vi "Withdrawal.vi"(8 "error in (no error)":errorcluster, 11 "ATM Controller in":refnum<class "ATM Controller.lvclass">) -> (0 "error out":errorcluster, 3 "ATM Controller out":refnum<class "ATM Controller.lvclass">)   [LabVIEW 2019, in "ATM Controller.lvlib" / "ATM Controller.lvclass"]
uses:
  ATM Controller.lvclass
  C:/Program Files (x86)/National Instruments/LabVIEW 2019/vi.lib/ActorFramework/Actor/Actor.lvclass
  <vilib>/ActorFramework/Actor/Actor.lvclass/Actor.ctl
  <vilib>/ActorFramework/Message Enqueuer/Message Enqueuer.lvclass/Message Enqueuer.ctl
  ATM Controller.lvclass/ATM Controller.ctl
  Message Name.ctl
  Simulated Configuration Database Actor/Configuration Database Actor Messages/Write Record Msg/Write Record Msg.lvclass/Write Record Msg.ctl
  ATM Controller Messages/Set ATM Message Msg/Set ATM Message Msg.lvclass/Set ATM Message Msg.ctl
  <vilib>/ActorFramework/Message Enqueuer/Init from Existing Queue.vi
  <vilib>/ActorFramework/Message Enqueuer/Enqueue.vi
  Simulated Configuration Database Actor/Configuration Database Actor Messages/Write Record Msg/Write Record Msg.lvclass
  C:/Program Files (x86)/National Instruments/LabVIEW 2019/vi.lib/ActorFramework/Message/Message.lvclass
  ATM Controller Messages/Set ATM Message Msg/Set ATM Message Msg.lvclass
  <vilib>/ActorFramework/Message Priority Queue/Priority Enqueue.vi
  <vilib>/ActorFramework/Message Enqueuer/Message Enqueuer.lvclass
  <vilib>/ActorFramework/Actor/Actor.lvclass
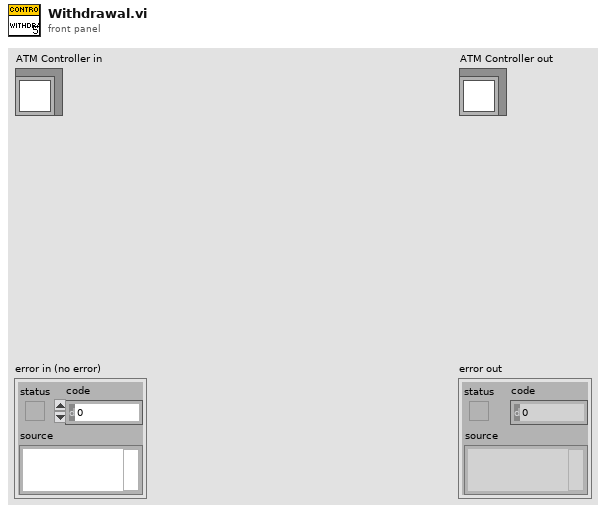
[diagram p1: front panel]
types:
  T1 = typedef "ATM Controller.lvlib/ATM Controller.lvclass/Message Name.ctl" = enum16{"Welcome", "Login", "Idle", "Invalid Login", "Terminate Session", "Deposit", "Withdrawal", "Fast Cash $50", "Withdrawal Failed", "Balance Inquiry"}
  T2 = typedef "Configuration Database Actor.lvlib/Configuration Database Actor.lvclass/Records -cluster.ctl" = cluster{"Account Number":i32, "First Name":string, "Last Name":string, "Balance":i32}
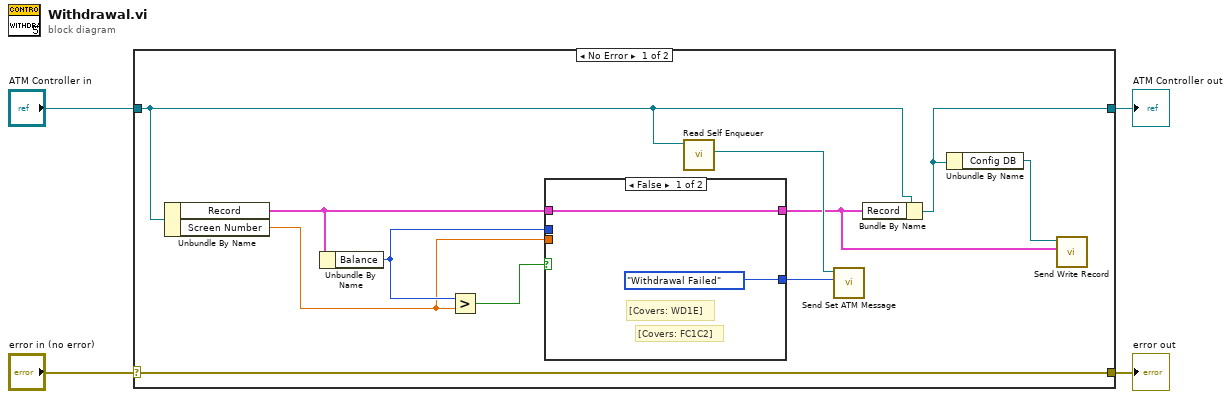
[diagram p0: block diagram]
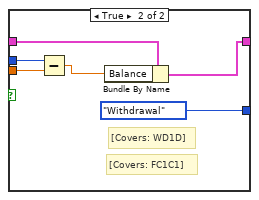
[diagram p2: hidden frame]
diagram:
  n1 = case shown="No Error" "error in (no error)" {
    selector: "error in (no error)" -> [w15 w25]
    tunnel: [w15 w25] -> w3
    tunnel: [w6 w24] -> w1
    tunnel: "ATM Controller in" -> [w10 w24]
    frame No Error {
      n2 = Unbundle By Name(w10) -> ("Record"=w12:T2, "Screen Number"=w8:dbl)
      n3 = Unbundle By Name(w12) -> ("Balance"=w9:i32)
      n4 = Greater?(x=w9, y=w8) -> (0:w14:bool)
      n5 = case shown="False" w14 {
        tunnel: [Message_Name."Withdrawal Failed" ("Message Name") Message_Name."Withdrawal" ("Message Name")] -> w13
        tunnel: w12 -> [w16 w22]
        tunnel: [w16 w18] -> w7
        tunnel: w9 -> [_ w21]
        tunnel: w8 -> [_ w20]
        frame False {
          # "[Covers: FC1C2]"
          # "[Covers: WD1E]"
        }
        frame True {
          # "[Covers: FC1C1]"
          # "[Covers: WD1D]"
          n6 = Subtract(x=w21, y=w20) -> (x-y=w19:dbl)
          n7 = Bundle By Name(cluster=w22, "Balance"=w19) -> (w18:T2)
        }
      }
      n8 = call <vilib>:"Read Self Enqueuer.vi"("Actor"=w10) -> ("Self Enqueuer"=w11:refnum<class "Message Enqueuer.lvclass">)  [unwired: 10 in]
      n9 = call "Send Set ATM Message.vi"("Message Name"=w13, "Message Enqueuer"=w11) -> ()  [unwired: 8 in, 2 out]
      n10 = Bundle By Name(cluster=w10, "Record"=w7) -> (w6:refnum<class "ATM Controller.lvclass">)
      n11 = Unbundle By Name(w6) -> ("Config DB"=w5:refnum<class "Message Enqueuer.lvclass">)
      n12 = call "Send Write Record.vi"("Record"=w7, "Message Enqueuer"=w5) -> ()  [unwired: 8 in, 2 out]
    }
    frame Error {
    }
  }
  "error out" <- w3
  "ATM Controller out" <- w1
